vi "Voronoi_Get Points Edges.vi"(10 "Edge Y":dbl[][](array[numeric]), 11 "Edge X":dbl[][](array[numeric])) -> (1 "Voronoi Edges":i32[][](array[numeric]), 2 "Voronoi Y":dbl[](array[numeric]), 3 "Voronoi X":dbl[](array[numeric]))   [LabVIEW 2020, in "NI_AAL_Geometry.lvlib"]
uses:
  <vilib>/Analysis/NI_AAL_Geometry.lvlib
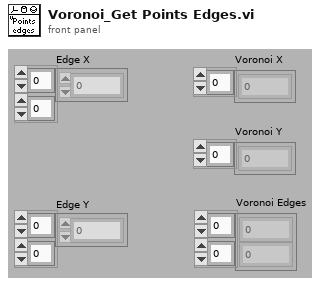
[diagram p1: front panel]
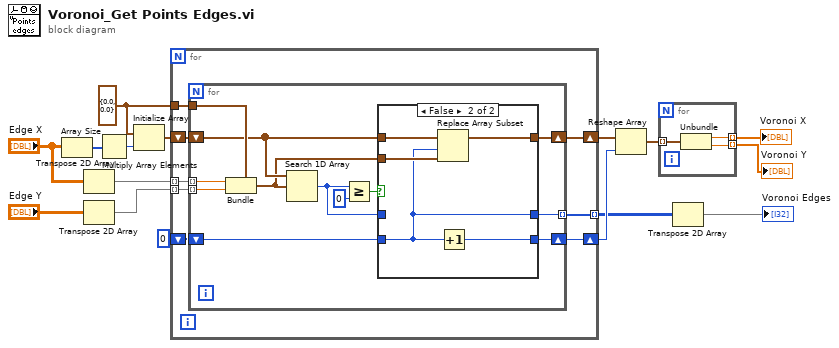
[diagram p0: block diagram]
diagram:
  w1 = cluster{dbl, dbl} {0.0, 0.0}
  n1 = Array Size(array="Edge X") -> (size(s)=w15:i32[])
  n2 = Transpose 2D Array(2D array="Edge X") -> (transposed array=w9:dbl[][])
  n3 = Transpose 2D Array(2D array="Edge Y") -> (transposed array=w7:dbl[][])
  n4 = Multiply Array Elements(1:w15) -> (0:w14:i32)
  n5 = Initialize Array(w1, w14) -> (w13:cluster{dbl, dbl}[])
  n6 = for {
    tunnel: w9 -> [w18] mode=indexing
    tunnel: w7 -> [w22] mode=indexing
    shift-right: [w17] -> w12
    shift-left: w13 -> [w23]
    tunnel: w1 -> [w24]
    shift-right: [w20] -> w11
    shift-left: 0 -> [w21]
    tunnel: [w19] -> w6 mode=indexing
    n7 = for {
      tunnel: w18 -> [w31] mode=indexing
      tunnel: w24 -> [w36]
      tunnel: w22 -> [w30] mode=indexing
      tunnel: [w26] -> w19 mode=indexing
      shift-right: [w25] -> w17
      shift-left: w23 -> [w35]
      shift-right: [w28] -> w20
      shift-left: w21 -> [w29]
      n8 = Bundle(cluster=w36, w31, w30) -> (w32:cluster{dbl, dbl})
      n9 = Search 1D Array(1D array=w35, element=w32) -> (index of element=w27:i32)  [unwired: 1 in]
      n10 = Greater Or Equal?(x=w27, y=0) -> (x >= y?=w33:bool)
      n11 = case shown="False" w33 {
        tunnel: [w39 w44] -> w25
        tunnel: w35 -> [w39 w43]
        tunnel: w32 -> [_ w42]
        tunnel: w29 -> [w38 w40]
        tunnel: [w38 w41] -> w28
        tunnel: w27 -> [w37 _]
        tunnel: [w37 w40] -> w26
        frame True {
        }
        frame False {
          n12 = Replace Array Subset(array=w43, new element=w42, index=w40) -> (w44:cluster{dbl, dbl}[])
          n13 = Increment(x=w40) -> (x+1=w41:i32)
        }
      }
    }
  }
  n14 = Reshape Array(w12, w11) -> (w4:cluster{dbl, dbl}[])
  n15 = for {
    tunnel: w4 -> [w47] mode=indexing
    tunnel: [w46] -> w3 mode=indexing
    tunnel: [w45] -> w2 mode=indexing
    n16 = Unbundle(w47) -> (w46:dbl, w45:dbl)
  }
  "Voronoi X" <- w3
  "Voronoi Y" <- w2
  n17 = Transpose 2D Array(2D array=w6) -> (transposed array=→"Voronoi Edges":i32[][])
